vi "Constructor.vi"(4 "TimeZoneInfoId":string, 5 "ProcessRunStartTime":timestamp, 6 "ProcessRunStatus":T1=enum."NOT_COMPLETED", 7 "ProductFullName":string, 8 "error in":errorcluster, 9 "ProductUnitIdentifier":string, 10 "ProcessFullName":string, 11 "Name":string) -> (0 "error out":errorcluster, 3 "ProcessRun out":refnum<class "ProcessRun.lvclass">)   [LabVIEW 2021, in "ProligentXMLGenerator.lvlib" / "ProcessRun.lvclass"]
uses:
  ProcessRun.lvclass
  ProcessRun.lvclass/ProcessRun.ctl
  Base/DateTime/DateTime.lvclass
  Base/ProcessFullName/ProcessFullName.lvclass
  Base/ExecutionStatus/ExecutionStatus.lvclass
  OperationRun/OperationRun.lvclass
  Base/NonEmptyString_50/NonEmptyString_50.lvclass
  Base/FullName/FullName.lvclass
  Data.ctl
  Base/NonEmptyString_64/NonEmptyString_64.lvclass
  Base/Guid/Guid.lvclass
  OperationCycle/OperationCycle.lvclass
  Failure/FailureReference/FailureReference.lvclass
  Model/CustomData/CustomData.lvclass
  Base/ExecutionStatus/Value.ctl
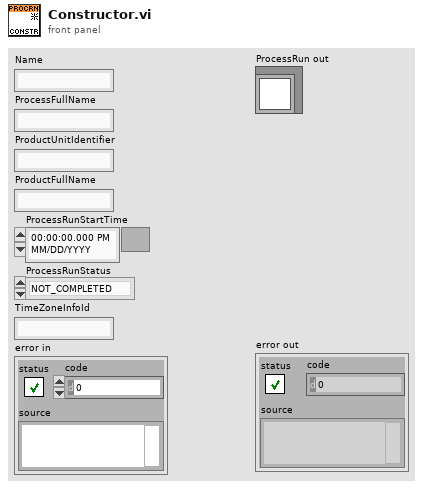
[diagram p1: front panel]
types:
  T1 = typedef "ProligentXMLGenerator.lvlib/ExecutionStatus.lvclass/Value.ctl" = enum16{"PASS", "FAIL", "NOT_COMPLETED", "ABORTED"}
  T2 = typedef "ProligentXMLGenerator.lvlib/ProcessRun.lvclass/Data.ctl" = cluster{"Name":string, "OperationRuns":refnum<class "OperationRun.lvclass">[], "OperationCycles":refnum<class "OperationCycle.lvclass">[], "FailureReferences":refnum<class "FailureReference.lvclass">[], "CustomData":refnum<class "CustomData.lvclass">, "ProcessRunId":refnum<class "Guid.lvclass">, "ProcessFullName":refnum<class "ProcessFullName.lvclass">, "ProcessVersion":refnum<class "NonEmptyString_64.lvclass">, "ProductUnitIdentifier":refnum<class "NonEmptyString_50.lvclass">, "ProductFullName":refnum<class "FullName.lvclass">, "ProcessRunStatus":refnum<class "ExecutionStatus.lvclass">, "ProcessRunStartTime":refnum<class "DateTime.lvclass">, "ProcessRunEndTime":refnum<class "DateTime.lvclass">, "ProcessMode":refnum<class "NonEmptyString_64.lvclass">, "TimeZoneInfoId":string}
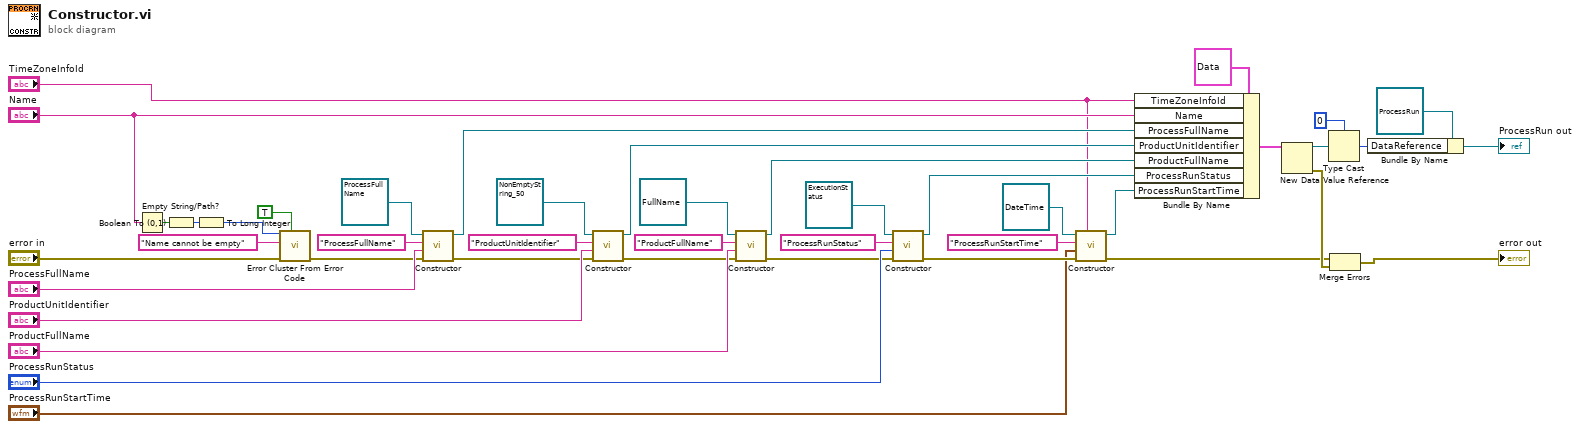
[diagram p0: block diagram]
diagram:
  n1 = Empty String/Path?(string/path="Name") -> (empty?=w26:bool)
  n2 = Boolean To (0,1)(Boolean=w26) -> (0, 1=w25:i16)
  n3 = To Long Integer(number=w25) -> (32bit integer=w24:i32)
  n4 = call <vilib>:"Error Cluster From Error Code.vi"("show call chain? (False)"=TRUE, "error in (no error)"="error in", "error message (\"\")"="Name cannot be empty" ("error message (\"\")"), "error code (0)"=w24) -> ("error out"=w20:errorcluster)  [unwired: 5 in]
  n5 = call-dynamic "Constructor.vi"("error in"=w20, "Value"="ProcessFullName", "Name"="ProcessFullName", "String in"=refnum<class "ProcessFullName.lvclass"> refnum ("ProligentResultProcessor:ProcessFullName")) -> ("error out"=w15:errorcluster, "String out"=w21:refnum<class "ProcessFullName.lvclass">)  [unwired: 6 in]
  n6 = call-dynamic "Constructor.vi"("error in"=w15, "Value"="ProductUnitIdentifier", "Name"="ProductUnitIdentifier", "String in"=refnum<class "NonEmptyString_50.lvclass"> refnum ("ProligentResultProcessor:NonEmptyString_65")) -> ("error out"=w7:errorcluster, "String out"=w14:refnum<class "NonEmptyString_50.lvclass">)  [unwired: 6 in]
  n7 = call-dynamic "Constructor.vi"("error in"=w7, "Value"="ProductFullName", "Name"="ProductFullName", "String in"=refnum<class "FullName.lvclass"> refnum ("ProligentResultProcessor:NonEmptyString_65")) -> ("error out"=w6:errorcluster, "String out"=w5:refnum<class "FullName.lvclass">)  [unwired: 6 in]
  n8 = call-dynamic "Constructor.vi"("error in"=w6, "Value"="ProcessRunStatus", "Name"="ProcessRunStatus", "ExecutionStatus in"=refnum<class "ExecutionStatus.lvclass"> refnum ("ProligentResultProcessor:ExecutionStatus")) -> ("error out"=w13:errorcluster, "ExecutionStatus out"=w10:refnum<class "ExecutionStatus.lvclass">)  [unwired: 6 in]
  n9 = call-dynamic "Constructor.vi"("TimeZoneInfoId"="TimeZoneInfoId", "error in"=w13, "Value"="ProcessRunStartTime", "Name"="ProcessRunStartTime", "DateTime in"=refnum<class "DateTime.lvclass"> refnum) -> ("error out"=w19:errorcluster, "DateTime out"=w28:refnum<class "DateTime.lvclass">)  [unwired: 5 in]
  n10 = Bundle By Name(cluster=T2 {"Name"="", "OperationRuns"=[], "OperationCycles"=[], "FailureReferences"=[], "CustomData"=refnum, "ProcessRunId"=refnum, "ProcessFullName"=refnum, "ProcessVersion"=refnum, "ProductUnitIdentifier"=refnum, "ProductFullName"=refnum, "ProcessRunStatus"=refnum, "ProcessRunStartTime"=refnum, "ProcessRunEndTime"=refnum, "ProcessMode"=refnum, "TimeZoneInfoId"=""} ("Data"), "TimeZoneInfoId"="TimeZoneInfoId", "Name"="Name", "ProcessFullName"=w21, "ProductUnitIdentifier"=w14, "ProductFullName"=w5, "ProcessRunStatus"=w10, "ProcessRunStartTime"=w28) -> (w33:T2)
  n11 = New Data Value Reference(data value=w33) -> (data value reference=w32:refnum<data-value>, error out=w29:errorcluster)  [unwired: 1 in]
  n12 = Type Cast(type=u64 0, x=w32) -> (*(type *) &x=w30:u64)
  n13 = Merge Errors(w19, w29) -> (→"error out":errorcluster)
  n14 = Bundle By Name(cluster=refnum<class "ProcessRun.lvclass"> refnum ("ProligentResultProcessor:ProcessRun"), "DataReference"=w30) -> (→"ProcessRun out":refnum<class "ProcessRun.lvclass">)
